vi "DIOArrayChange.vi"(3 "Changed DIO Tydef":T1, 5 "Experiment State in":T2={"error"={"status"=FALSE, "code"=0, "source"=""}, "Digitizer DAQmx Tasks"={"TaskArray"=[]}, "DAQ Settings"={"Channel Settings"=[], "Card Settings"=[]}, "Synchronization Settings"={"Synchronizer 0"="", "source terminal"="", "Synchronizer 1"="PXI1Slot2"}, "DAQ Data"=[], "Next Shot#"="", "System Message"="", "User Shot Notes"="", "Timing Settings"={"Timing Card Settings"=[], "Timing Channel Settings"=[]}, "Timing Tasks"={"TaskArray"=[]}, "Tree"="", "Time Card/Channels"=[], "DAQ Card/Channels"=[], "Program Version"="", "RIO Settings"={"Channel Settings"=[], "Card Settings"=[]}, "RIO References"={"Reference Array"=[]}, "RIO Data"={"RIO Deleaved Data"=[], "Raw Readout"=[]}, "RIO Card/Channels"=[3, 8], "DIO Channels"=0, "DIO Settings"={"DIO Channel Array"=[]}, "Global Settings"={"Initial Background Values"={"Reference Shot #"=0.0, "Background pressure [Torr]"=0.0, "Cryo temp [V]"=0.0, "Cryo temp [K]"=0.0, "Cryotemp Calibration File"=path ""}, "Gas Puffing"={"Gas A type"="N", "Gas B type"="N", "Gas C type"="N", "Gas A pressure [psi]"=0.0, "Gas B pressure [psi]"=0.0, "Gas C pressure [psi]"=0.0, "Innner Electrode"="", "Middle Electrode"="", "Outer Electrode"="", "Gas A bottle pressure [psi]"=0.0, "Gas B bottle pressure [psi]"=0.0, "Gas C bottle pressure [psi]"=0.0}, "PSU Voltages"={"Bias1 Voltage [V]"=0.0, "Bias2 Voltage [V]"=0.0, "PSU1 Voltage [V]"=0.0, "Puff-PSU1 CH1 Voltage [V]"=0.0, "Puff-PSU1 CH2 Voltage [V]"=0.0, "Puff-PSU1 CH3 Voltage [V]"=0.0}, "Scope Details"={"CH1"="", "CH2"="", "CH3"="", "CH4"="", "CH1 Ground State"="Grounded", "CH2 Ground State"="Grounded", "CH3 Ground State"="Grounded", "CH4 Ground State"="Grounded"}}, "Calibrations"={"CryoTemp"={"Comment"="", "X"=[], "Y"=[]}, "PSU2 Tach"={"Comment"="", "X"=[], "Y"=[]}, "PSU3 Tach"={"Comment"="", "X"=[], "Y"=[]}}, "Tach Tasks"={"PSU2 task"="", "PSU3 task"=""}, "PSU2 Tachometer Controls"={"PSU2 Tach Calibration"=path "Z:/Data/Calibration/Tachometer", "PSU2 charging Voltage [kV]"=0.0, "PSU2 Counter"=""}, "PSU3 Tachometer Controls"={"PSU3 Tach Calibration"=path "Z:/Data/Calibration/Tachometer/PSU3_TachCalibration.csv", "PSU3 charging Voltage [kV]"=0.0, "PSU3 Counter"=""}, "PSU2 DIO channels"={"Charge relay DIO"="DAQ0/port0/line3", "Dump relay DIO"="DAQ0/port0/line4", "HV Arm DIO"="DAQ0/port0/line5", "HV On DIO"="DAQ0/port0/line6"}, "PSU3 DIO channels"={"Charge relay DIO"="DAQ0/port0/line3", "Dump relay DIO"="DAQ0/port0/line4", "HV Arm DIO"="DAQ0/port0/line5", "HV On DIO"="DAQ0/port0/line6"}, "PSU2 Reverse Tachometer Controls"={"PSU2 RevTach Calibration"=path "Z:/Data/Calibration/Reverse Tachometer/PSU2_RevTachCalibration.csv", "PSU2 bank Voltage [kV]"=0.0, "PSU2 RevTach Counter"=""}, "PSU3 Reverse Tachometer Controls"={"PSU3 RevTach Calibration"=path "Z:/Data/Calibration/Reverse Tachometer/PSU3_RevTachCalibration.csv", "PSU3 bank Voltage [kV]"=0.0, "PSU3 RevTach Counter"=""}} {"Global Settings"."Initial Background Values"."Cryo temp [K]" format="%#_4g"; "RIO Settings"."Card Settings"."Sample Rate" format="%#_3p"; "Timing Settings"."Timing Channel Settings"."FrontPanelTime" format="%.3p"; "Timing Settings"."Timing Channel Settings"."Pulse width (s)" format="%.3p"; "Timing Settings"."Timing Channel Settings"."Delay (s)" format="%.3p"; "DAQ Settings"."Card Settings"."Global Edge Type" items=["Rising"=10280, "Falling"=10171]; "DAQ Settings"."Card Settings"."Sample Rate" format="%#_3p"}) -> (2 "Experiment State out":T2={"error"={"status"=FALSE, "code"=0, "source"=""}, "Digitizer DAQmx Tasks"={"TaskArray"=[]}, "DAQ Settings"={"Channel Settings"=[], "Card Settings"=[]}, "Synchronization Settings"={"Synchronizer 0"="", "source terminal"="", "Synchronizer 1"="PXI1Slot2"}, "DAQ Data"=[], "Next Shot#"="", "System Message"="", "User Shot Notes"="", "Timing Settings"={"Timing Card Settings"=[], "Timing Channel Settings"=[]}, "Timing Tasks"={"TaskArray"=[]}, "Tree"="", "Time Card/Channels"=[], "DAQ Card/Channels"=[], "Program Version"="", "RIO Settings"={"Channel Settings"=[], "Card Settings"=[]}, "RIO References"={"Reference Array"=[]}, "RIO Data"={"RIO Deleaved Data"=[], "Raw Readout"=[]}, "RIO Card/Channels"=[3, 8], "DIO Channels"=0, "DIO Settings"={"DIO Channel Array"=[]}, "Global Settings"={"Initial Background Values"={"Reference Shot #"=0.0, "Background pressure [Torr]"=0.0, "Cryo temp [V]"=0.0, "Cryo temp [K]"=0.0, "Cryotemp Calibration File"=path ""}, "Gas Puffing"={"Gas A type"="N", "Gas B type"="N", "Gas C type"="N", "Gas A pressure [psi]"=0.0, "Gas B pressure [psi]"=0.0, "Gas C pressure [psi]"=0.0, "Innner Electrode"="", "Middle Electrode"="", "Outer Electrode"="", "Gas A bottle pressure [psi]"=0.0, "Gas B bottle pressure [psi]"=0.0, "Gas C bottle pressure [psi]"=0.0}, "PSU Voltages"={"Bias1 Voltage [V]"=0.0, "Bias2 Voltage [V]"=0.0, "PSU1 Voltage [V]"=0.0, "Puff-PSU1 CH1 Voltage [V]"=0.0, "Puff-PSU1 CH2 Voltage [V]"=0.0, "Puff-PSU1 CH3 Voltage [V]"=0.0}, "Scope Details"={"CH1"="", "CH2"="", "CH3"="", "CH4"="", "CH1 Ground State"="Grounded", "CH2 Ground State"="Grounded", "CH3 Ground State"="Grounded", "CH4 Ground State"="Grounded"}}, "Calibrations"={"CryoTemp"={"Comment"="", "X"=[], "Y"=[]}, "PSU2 Tach"={"Comment"="", "X"=[], "Y"=[]}, "PSU3 Tach"={"Comment"="", "X"=[], "Y"=[]}}, "Tach Tasks"={"PSU2 task"="", "PSU3 task"=""}, "PSU2 Tachometer Controls"={"PSU2 Tach Calibration"=path "Z:/Data/Calibration/Tachometer", "PSU2 charging Voltage [kV]"=0.0, "PSU2 Counter"=""}, "PSU3 Tachometer Controls"={"PSU3 Tach Calibration"=path "Z:/Data/Calibration/Tachometer/PSU3_TachCalibration.csv", "PSU3 charging Voltage [kV]"=0.0, "PSU3 Counter"=""}, "PSU2 DIO channels"={"Charge relay DIO"="DAQ0/port0/line3", "Dump relay DIO"="DAQ0/port0/line4", "HV Arm DIO"="DAQ0/port0/line5", "HV On DIO"="DAQ0/port0/line6"}, "PSU3 DIO channels"={"Charge relay DIO"="DAQ0/port0/line3", "Dump relay DIO"="DAQ0/port0/line4", "HV Arm DIO"="DAQ0/port0/line5", "HV On DIO"="DAQ0/port0/line6"}, "PSU2 Reverse Tachometer Controls"={"PSU2 RevTach Calibration"=path "Z:/Data/Calibration/Reverse Tachometer/PSU2_RevTachCalibration.csv", "PSU2 bank Voltage [kV]"=0.0, "PSU2 RevTach Counter"=""}, "PSU3 Reverse Tachometer Controls"={"PSU3 RevTach Calibration"=path "Z:/Data/Calibration/Reverse Tachometer/PSU3_RevTachCalibration.csv", "PSU3 bank Voltage [kV]"=0.0, "PSU3 RevTach Counter"=""}} {"Global Settings"."Initial Background Values"."Cryo temp [K]" format="%#_4g"; "RIO Settings"."Card Settings"."Sample Rate" format="%#_3p"; "Timing Settings"."Timing Channel Settings"."FrontPanelTime" format="%.3p"; "Timing Settings"."Timing Channel Settings"."Pulse width (s)" format="%.3p"; "Timing Settings"."Timing Channel Settings"."Delay (s)" format="%.3p"; "DAQ Settings"."Card Settings"."Global Edge Type" items=["Rising"=10280, "Falling"=10171]; "DAQ Settings"."Card Settings"."Sample Rate" format="%#_3p"})   [LabVIEW 2014]
doc: "Handle DIO changes identified in the producer."
uses:
  Controls/ExperimentStateCluster.ctl
  Controls/DigitizerSettingsChannelSettings.ctl
  Controls/DigitizerSettingsCardSettingsArray.ctl
  Controls/DigitizerSettingsCardSettings.ctl
  Controls/TimingSettings.ctl
  Controls/TimingCardSettings.ctl
  Controls/TimingChannelSettings.ctl
  Controls/RIOSettingsExperimentStateCluster.ctl
  Controls/RIOChannelSettingsArrayExperimentStateCluster.ctl
  Controls/RIOSettingsChannelSettings.ctl
  Controls/RIOSettingsCardSettingsArray.ctl
  Controls/RIOSettingsCardSettings.ctl
  <vilib>/userdefined/High Color/nirio_resource_hc.ctl
  Controls/RIOData.ctl
  Controls/DIOChannel.ctl
  Controls/Global Settings/GlobalSettings.ctl
  Controls/Global Settings/InitialBackgroundValues.ctl
  Controls/Global Settings/GasPuffing.ctl
  Controls/Global Settings/PSUVoltages.ctl
  Controls/Global Settings/ScopeDetails.ctl
  Controls/Calibrations/Calibrations.ctl
  Controls/Calibrations/CryoTemoCalibration.ctl
  Controls/Calibrations/PSU2TachCalibration.ctl
  Controls/Calibrations/PSU3TachCalibration.ctl
  Controls/TachTasks.ctl
  Controls/PSU2TachometerControls.ctl
  Controls/PSU3TachometerControls.ctl
  Controls/PSU2DIOChannels.ctl
  Controls/PSU3DIOChannels.ctl
  Controls/PSU2ReverseTachometerControls.ctl
  Controls/PSU3ReverseTachometerControls.ctl
  Controls/ChangedDIOTypdef.ctl
  <vilib>/DAQmx/create/channels.llb/DAQmx Create Channel (DO-Digital Output).vi
  <vilib>/DAQmx/write.llb/DAQmx Write (Digital Bool 1Line 1Point).vi
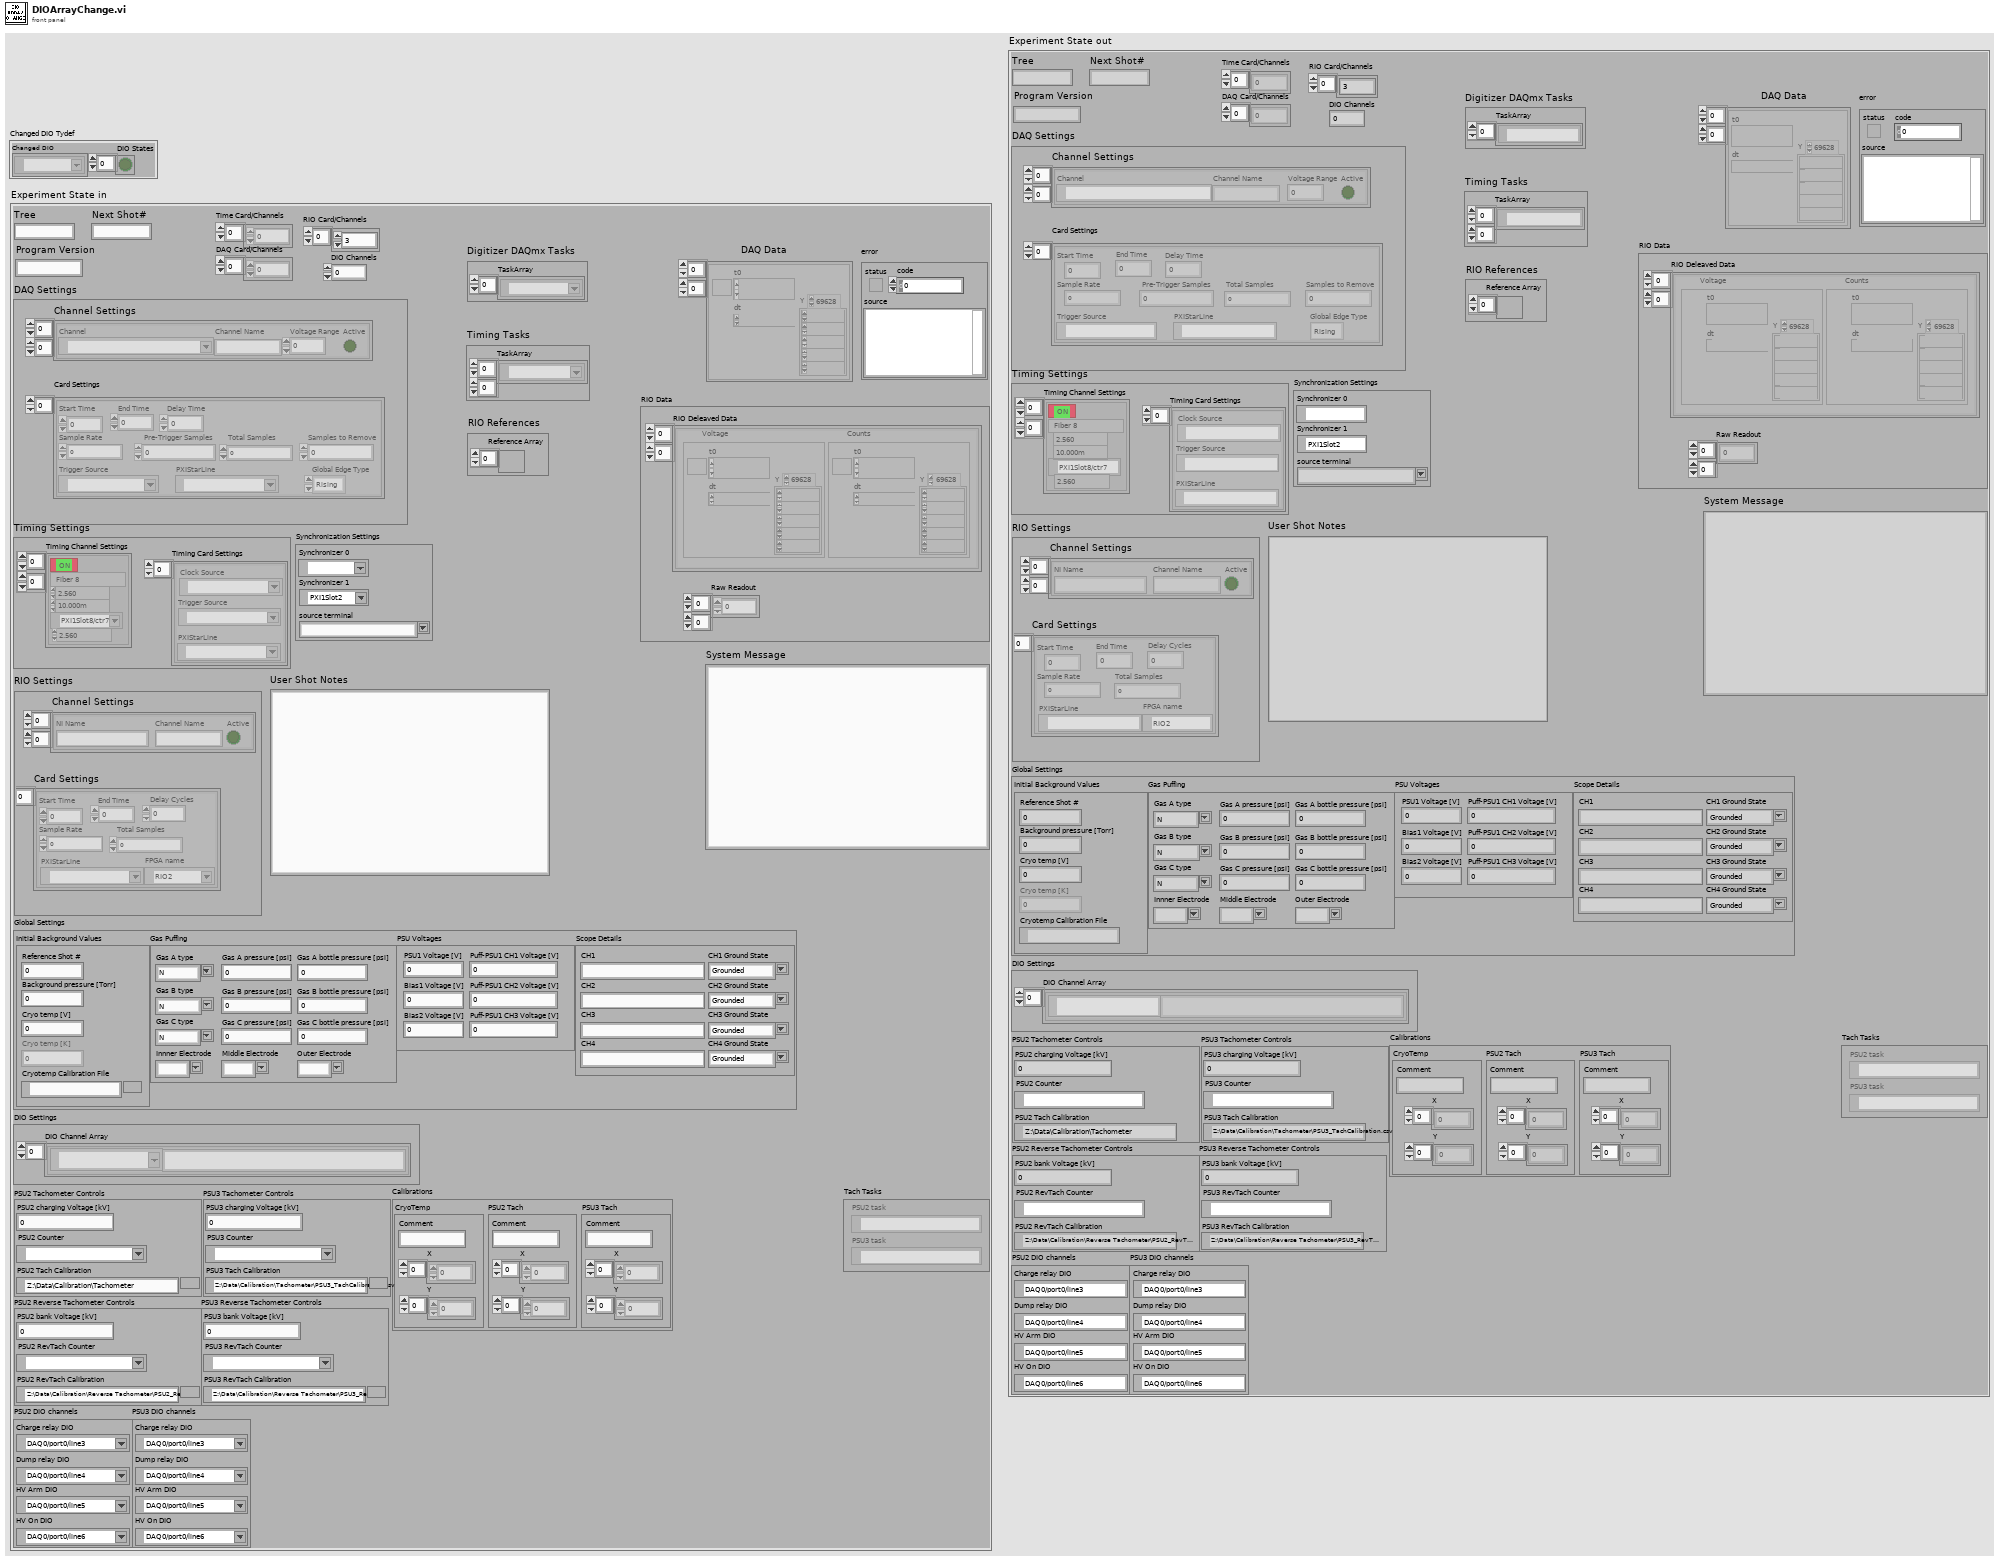
[diagram p1: front panel]
types:
  T1 = typedef "ChangedDIOTypdef.ctl" = cluster{"Changed DIO":tag[], "DIO States":bool[]}
  T2 = typedef "ExperimentStateCluster.ctl" = cluster{"error":errorcluster, "Digitizer DAQmx Tasks":cluster{"TaskArray":refnum<k21>[]}, "DAQ Settings":cluster{"Channel Settings":T3[][], "Card Settings":T4}, "Synchronization Settings":cluster{"Synchronizer 0":refnum<k15>, "source terminal":string, "Synchronizer 1":refnum<k15>}, "DAQ Data":waveform(dbl)[][], "Next Shot#":string, "System Message":string, "User Shot Notes":string, "Timing Settings":T6, "Timing Tasks":cluster{"TaskArray":refnum<k21>[][]}, "Tree":string, "Time Card/Channels":i32[], "DAQ Card/Channels":i32[], "Program Version":string, "RIO Settings":T9, "RIO References":cluster{"Reference Array":refnum<k20>[]}, "RIO Data":T15, "RIO Card/Channels":i32[], "DIO Channels":i32, "DIO Settings":cluster{"DIO Channel Array":T16[]}, "Global Settings":T17, "Calibrations":T22, "Tach Tasks":T26, "PSU2 Tachometer Controls":T27, "PSU3 Tachometer Controls":T28, "PSU2 DIO channels":T29, "PSU3 DIO channels":T30, "PSU2 Reverse Tachometer Controls":T31, "PSU3 Reverse Tachometer Controls":T32}
  T3 = typedef "DigitizerSettingsChannelSettings.ctl" = cluster{"Channel":tag, "Channel Name":string, "Voltage Range":dbl, "Active":bool}
  T4 = typedef "DigitizerSettingsCardSettingsArray.ctl" = T5[]
  T5 = typedef "DigitizerSettingsCardSettings.ctl" = cluster{"Start Time":dbl, "End Time":dbl, "Sample Rate":dbl, " Pre-Trigger Samples":u32, "Total Samples":i32, "Samples to Remove":u32, "Trigger Source":tag, "Global Edge Type":i32, "PXIStarLine":tag, "Delay Time":dbl}
  T6 = typedef "TimingSettings.ctl" = cluster{"Timing Card Settings":T7[], "Timing Channel Settings":T8[][]}
  T7 = typedef "TimingCardSettings.ctl" = cluster{"Trigger Source":tag, "Clock Source":tag, "PXIStarLine":tag}
  T8 = typedef "TimingChannelSettings.ctl" = cluster{"Delay (s)":dbl, "Pulse width (s)":dbl, "Active":bool, "Channel Name":string, "counter":tag, "FrontPanelTime":dbl}
  T9 = typedef "RIOSettingsExperimentStateCluster.ctl" = cluster{"Channel Settings":T10, "Card Settings":T12}
  T10 = typedef "RIOChannelSettingsArrayExperimentStateCluster.ctl" = T11[][]
  T11 = typedef "RIOSettingsChannelSettings.ctl" = cluster{"Channel Name":string, "Active":bool, "NI Name":string}
  T12 = typedef "RIOSettingsCardSettingsArray.ctl" = T13[]
  T13 = typedef "RIOSettingsCardSettings.ctl" = cluster{"Start Time":dbl, "End Time":dbl, "Sample Rate":dbl, "Total Samples":u64, "PXIStarLine":tag, "Delay Cycles":u64, "FPGA name":T14}
  T14 = typedef "nirio_resource_hc.ctl" = tag
  T15 = typedef "RIOData.ctl" = cluster{"RIO Deleaved Data":cluster{"Voltage":waveform(dbl), "Counts":waveform(i16)}[][], "Raw Readout":u64[][]}
  T16 = typedef "DIOChannel.ctl" = cluster{"Channel Name":string, "NI Name":tag}
  T17 = typedef "GlobalSettings.ctl" = cluster{"Initial Background Values":T18, "Gas Puffing":T19, "PSU Voltages":T20, "Scope Details":T21}
  T18 = typedef "InitialBackgroundValues.ctl" = cluster{"Reference Shot #":dbl, "Background pressure [Torr]":dbl, "Cryo temp [V]":dbl, "Cryo temp [K]":dbl, "Cryotemp Calibration File":path}
  T19 = typedef "GasPuffing.ctl" = cluster{"Gas A type":string, "Gas B type":string, "Gas C type":string, "Gas A pressure [psi]":dbl, "Gas B pressure [psi]":dbl, "Gas C pressure [psi]":dbl, "Innner Electrode":string, "Middle Electrode":string, "Outer Electrode":string, "Gas A bottle pressure [psi]":dbl, "Gas B bottle pressure [psi]":dbl, "Gas C bottle pressure [psi]":dbl}
  T20 = typedef "PSUVoltages.ctl" = cluster{"Bias1 Voltage [V]":dbl, "Bias2 Voltage [V]":dbl, "PSU1 Voltage [V]":dbl, "Puff-PSU1 CH1 Voltage [V]":dbl, "Puff-PSU1 CH2 Voltage [V]":dbl, "Puff-PSU1 CH3 Voltage [V]":dbl}
  T21 = typedef "ScopeDetails.ctl" = cluster{"CH1":string, "CH2":string, "CH3":string, "CH4":string, "CH1 Ground State":string, "CH2 Ground State":string, "CH3 Ground State":string, "CH4 Ground State":string}
  T22 = typedef "Calibrations.ctl" = cluster{"CryoTemp":T23, "PSU2 Tach":T24, "PSU3 Tach":T25}
  T23 = typedef "CryoTemoCalibration.ctl" = cluster{"Comment":string, "X":dbl[], "Y":dbl[]}
  T24 = typedef "PSU2TachCalibration.ctl" = cluster{"Comment":string, "X":dbl[], "Y":dbl[]}
  T25 = typedef "PSU3TachCalibration.ctl" = cluster{"Comment":string, "X":dbl[], "Y":dbl[]}
  T26 = typedef "TachTasks.ctl" = cluster{"PSU2 task":refnum<k21>, "PSU3 task":refnum<k21>}
  T27 = typedef "PSU2TachometerControls.ctl" = cluster{"PSU2 Tach Calibration":path, "PSU2 charging Voltage [kV]":dbl, "PSU2 Counter":tag}
  T28 = typedef "PSU3TachometerControls.ctl" = cluster{"PSU3 Tach Calibration":path, "PSU3 charging Voltage [kV]":dbl, "PSU3 Counter":tag}
  T29 = typedef "PSU2DIOChannels.ctl" = cluster{"Charge relay DIO":tag, "Dump relay DIO":tag, "HV Arm DIO":tag, "HV On DIO":tag}
  T30 = typedef "PSU3DIOChannels.ctl" = cluster{"Charge relay DIO":tag, "Dump relay DIO":tag, "HV Arm DIO":tag, "HV On DIO":tag}
  T31 = typedef "PSU2ReverseTachometerControls.ctl" = cluster{"PSU2 RevTach Calibration":path, "PSU2 bank Voltage [kV]":dbl, "PSU2 RevTach Counter":tag}
  T32 = typedef "PSU3ReverseTachometerControls.ctl" = cluster{"PSU3 RevTach Calibration":path, "PSU3 bank Voltage [kV]":dbl, "PSU3 RevTach Counter":tag}
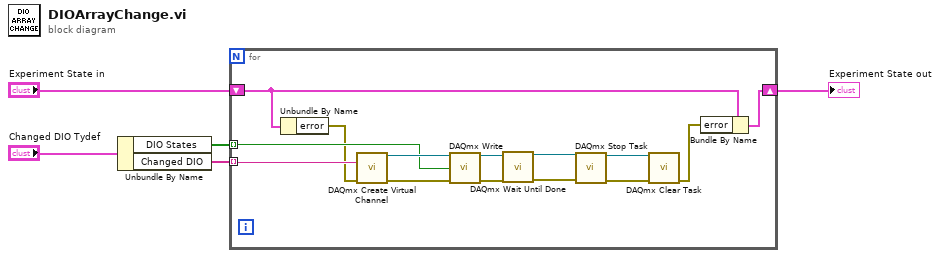
[diagram p0: block diagram]
diagram:
  n1 = Unbundle By Name("Changed DIO Tydef") -> ("DIO States"=w1:bool[], "Changed DIO"=w4:tag[])
  n2 = for {
    tunnel: w4 -> [w15] mode=indexing
    tunnel: w1 -> [w13] mode=indexing
    shift-right: [w7] -> w2
    shift-left: "Experiment State in" -> [w6]
    n3 = Unbundle By Name(w6) -> ("error"=w9:errorcluster)
    n4 = call-poly <vilib>:"DAQmx Create Virtual Channel.vi"("lines"=w15, "error in"=w9) -> ("task out"=w14:refnum<k21>, "error out"=w19:errorcluster)  [unwired: 12 in]
    n5 = call-poly <vilib>:"DAQmx Write.vi"("task/channels in"=w14, "data"=w13, "error in"=w19) -> ("task out"=w12:refnum<k21>, "error out"=w18:errorcluster)  [unwired: 1 in, 10 out]
    n6 = call <vilib>:"DAQmx Wait Until Done.vi"("task/channels in"=w12, "error in"=w18) -> ("task out"=w11:refnum<k21>, "error out"=w17:errorcluster)  [unwired: 12 in]
    n7 = call <vilib>:"DAQmx Stop Task.vi"("task/channels in"=w11, "error in"=w17) -> ("task out"=w10:refnum<k21>, "error out"=w16:errorcluster)  [unwired: 12 in]
    n8 = call <vilib>:"DAQmx Clear Task.vi"("task in"=w10, "error in"=w16) -> ("error out"=w8:errorcluster)  [unwired: 13 in]
    n9 = Bundle By Name(cluster=w6, "error"=w8) -> (w7:T2)
  }
  "Experiment State out" <- w2
